vi "crop_image_for splitting.vi"(11 "Image in":T1) -> (3 "Image out":T1)   [LabVIEW 2024]
uses:
  <vilib>/vision/Image Controls.llb/IMAQ Image.ctl
  <vilib>/Analysis/baseanly.llb/Mean (DBL).vi
  <vilib>/Analysis/NI_AALBase.lvlib
  <vilib>/vision/NI_Vision_Development_Module.lvlib
panel:
  in  "Intensity Threshold":i32=100
  in  "Number of rakes":i32=10
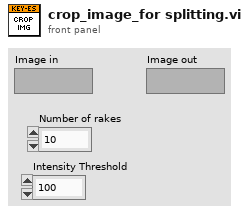
[diagram p1: front panel]
types:
  T1 = typedef "IMAQ Image.ctl" = refnum<image>
  T2 = typedef "Image Type" = u32
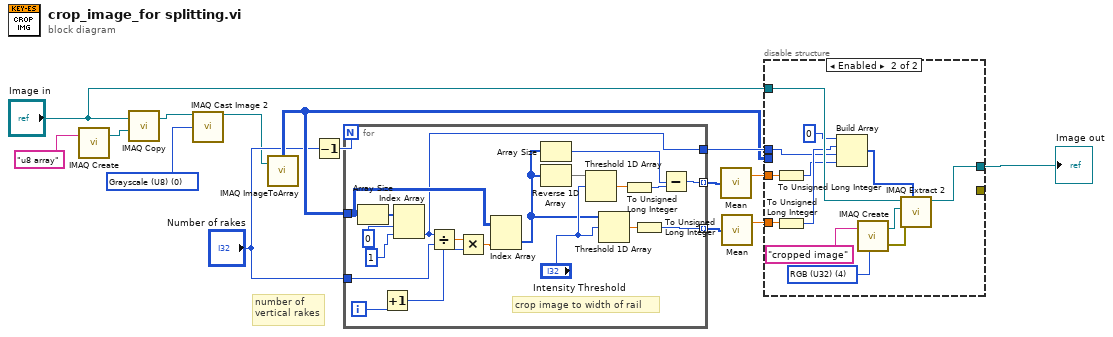
[diagram p0: block diagram]
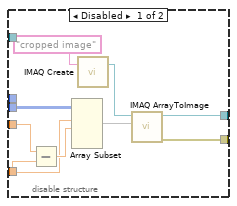
[diagram p2: hidden frame]
diagram:
  w1 = T2 0 items=["Grayscale (U8)", "Grayscale (I16)", "Grayscale (SGL)", "Complex (CSG)", "RGB (U32)", "HSL (U32)", "RGB (U64)", "Grayscale (U16)"] ("Image Type")
  # "number of\nvertical rakes"
  n1 = call "IMAQ Create"("Image Name"="u8 array") -> ("New Image"=w4:T1)  [unwired: 4 in, 1 out]
  n2 = call "IMAQ Copy"("Image Dst"=w4, "Image Src"="Image in") -> ("Image Dst Out"=w3:T1)  [unwired: 4 in, 1 out]
  n3 = call "IMAQ Cast Image 2"("Image Src"=w3, "Image Type"=w1) -> ("Image Dst Out"=w2:T1)  [unwired: 12 in, 1 out]
  n4 = call "IMAQ ImageToArray"("Image"=w2) -> ("Image Pixels (U8)"=w13:u8[][])  [unwired: 3 in, 4 out]
  n5 = Decrement(x="Number of rakes") -> (x-1=w8:i32)
  n6 = for {
    N: w8 -> [_]
    tunnel: w13 -> [w29]
    tunnel: "Number of rakes" -> [w34]
    tunnel: [w18] -> w10 mode=indexing
    tunnel: [w21] -> w9 mode=indexing
    tunnel: [w16] -> w14
    i -> [w27]
    # "crop image to width of rail"
    n7 = Array Size(array=w29) -> (size(s)=w30:i32[])
    n8 = Increment(x=w27) -> (x+1=w26:i32)
    n9 = Index Array(array=w30, index #1=0 ("index"), index #2=1 ("index")) -> (element #2=w16:i32)  [unwired: 1 out]
    n10 = Divide(x=w16, y=w34) -> (x/y=w33:dbl)
    n11 = Multiply(x=w33, y=w26) -> (x*y=w28:dbl)
    n12 = Index Array(array=w29, index (col)=w28) -> (element=w20:u8[])  [unwired: 1 in]
    n13 = Array Size(array=w20) -> (size(s)=w17:i32)
    n14 = Reverse 1D Array(array=w20) -> (reversed array=w24:u8[])
    n15 = Threshold 1D Array(2:"Intensity Threshold", 3:w24) -> (0:w22:dbl)  [unwired: 1 in]
    n16 = Threshold 1D Array(2:"Intensity Threshold", 3:w20) -> (0:w25:dbl)  [unwired: 1 in]
    n17 = To Unsigned Long Integer(number=w22) -> (unsigned 32bit integer=w19:u32)
    n18 = To Unsigned Long Integer(number=w25) -> (unsigned 32bit integer=w21:u32)
    n19 = Subtract(x=w17, y=w19) -> (x-y=w18:u32)
  }
  n20 = call-poly <vilib>:"Mean.vi"("X"=w10) -> ("mean"=w11:dbl)  [unwired: 1 out]
  n21 = call-poly <vilib>:"Mean.vi"("X"=w9) -> ("mean"=w12:dbl)  [unwired: 1 out]
  n22 = disable-structure shown="Enabled" {
    disable-tunnel: w11 -> [w43 w54]
    disable-tunnel: w12 -> [w41 w55]
    disable-tunnel: [w40 _] -> _
    disable-tunnel: [w37 w48] -> w15
    disable-tunnel: w13 -> [w36 _]
    disable-tunnel: "Image in" -> [_ w56]
    disable-tunnel: w14 -> [_ w51]
    frame Disabled {
      n23 = Subtract(x=w43, y=w41) -> (x-y=w42:dbl)
      n24 = Array Subset(array=w36, index (row)=w41, length (row)=w42) -> (w35:u8[][])  [unwired: 2 in]
      n25 = call "IMAQ Create"("Image Name"="cropped image") -> ("New Image"=w38:T1)  [unwired: 4 in, 1 out]
      n26 = call "IMAQ ArrayToImage"("Image Pixels (U8)"=w35, "Image"=w38) -> ("error out"=w40:errorcluster, "Image Out"=w37:T1)  [unwired: 8 in]
    }
    frame Enabled {
      w44 = T2 4 items=["Grayscale (U8)", "Grayscale (I16)", "Grayscale (SGL)", "Complex (CSG)", "RGB (U32)", "HSL (U32)", "RGB (U64)", "Grayscale (U16)"] ("Image Type")
      n27 = To Unsigned Long Integer(number=w54) -> (unsigned 32bit integer=w50:u32)
      n28 = To Unsigned Long Integer(number=w55) -> (unsigned 32bit integer=w52:u32)
      n29 = Build Array(0, w52, w51, w50) -> (w49:u32[])
      n30 = call "IMAQ Create"("Image Name"="cropped image", "Image Type"=w44) -> ("New Image"=w47:T1, "error out"=w46:errorcluster)  [unwired: 3 in]
      n31 = call "IMAQ Extract 2"("Optional Rectangle"=w49, "error in (no error)"=w46, "Image Dst"=w47, "Image Src"=w56) -> ("Image Dst Out"=w48:T1)  [unwired: 6 in, 1 out]
    }
  }
  "Image out" <- w15
